vi "Report Pump State.vi"(8 "error in (no error)":errorcluster, 10 "Pump State":bool, 11 "Evaporative Cooler in":refnum<class "Evaporative Cooler.lvclass">) -> (0 "error out":errorcluster)   [LabVIEW 2018, in "Evaporative Cooler.lvlib" / "Evaporative Cooler.lvclass"]
doc: "Sends a message to the controller reporting the state of the pump (on or off)."
uses:
  Evaporative Cooler.lvclass
  C:/GitClones/LGP5-Resources/Frameworks/Actor Framework/Feedback Evaporative Cooler/Cooler/Cooler/Cooler.lvclass
  <vilib>/ActorFramework/Message Enqueuer/Message Enqueuer.lvclass
  Cooler/Cooler/Cooler.lvclass/Cooler.ctl
  Evaporative Cooler Controller/Update Pump State Msg/Update Pump State Msg.lvclass/Update Pump State Msg.ctl
  <vilib>/ActorFramework/Message Enqueuer/Message Enqueuer.lvclass/Message Enqueuer.ctl
  <vilib>/ActorFramework/Message Enqueuer/Enqueue.vi
  Evaporative Cooler Controller/Update Pump State Msg/Update Pump State Msg.lvclass
  C:/Program Files (x86)/National Instruments/LabVIEW 2018/vi.lib/ActorFramework/Message/Message.lvclass
  <vilib>/ActorFramework/Message Priority Queue/Priority Enqueue.vi
  Cooler/Cooler/Cooler.lvclass
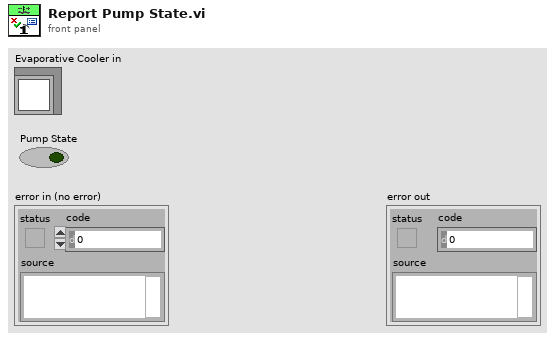
[diagram p1: front panel]
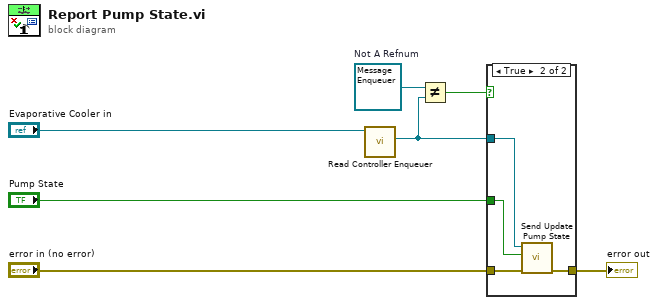
[diagram p0: block diagram]
diagram:
  w2 = refnum<class "Message Enqueuer.lvclass"> refnum  # Not A Refnum
  n1 = call "Read Controller Enqueuer.vi"("Cooler"="Evaporative Cooler in") -> ("Controller Enqueuer"=w3:refnum<class "Message Enqueuer.lvclass">)  [unwired: 10 in]
  n2 = Not Equal?(x=w2, y=w3) -> (x != y?=w1:bool)
  n3 = case shown="True" w1 {
    tunnel: "Pump State" -> [_ w12]
    tunnel: [w8 w11] -> w5
    tunnel: w3 -> [_ w10]
    tunnel: "error in (no error)" -> [w8 w9]
    frame False {
    }
    frame True {
      n4 = call "Send Update Pump State.vi"("error in (no error)"=w9, "Pump on?"=w12, "Message Enqueuer"=w10) -> ("error out"=w11:errorcluster)  [unwired: 8 in]
    }
  }
  "error out" <- w5
